vi "5492_SpitButton.vi"() -> ()   [LabVIEW 2017]
panel:
  in  "Spit Button":bool
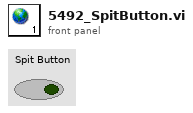
[diagram p1: front panel]
diagram:
